vi "SGDRegressor.vi"(8 "error in":errorcluster) -> (0 "error out":errorcluster, 3 "out":refnum<class "SGDRegressor.lvclass">)   [LabVIEW 2020]
doc: "Linear model fitted by minimizing a regularized empirical loss with SGD\n\n SGD stands for Stochastic Gradient Descent: the gradient of the loss is\n estimated each sample at a time and the model is updated along the way with\n a decreasing strength schedule (aka learning rate).\n\n The regularizer is a penalty added to the loss function that shrinks model\n parameters towards the zero vector using either the squared euclidean norm\n L2 or the absolute norm L1 or a combination of both (Elastic Net). If the\n parameter update crosses the 0.0 value because of the regularizer, the\n update is truncated to 0.0 to allow for learning sparse models and achieve\n online feature selection.\n\n This implementation works with data represented as dense numpy arrays of\n floating point values for the features.\n\n Read more in the :ref:`User Guide <sgd>`.\n\n Parameters\n ----------\n loss : str, default='squared_loss'\n The loss function to be used. The possible values are 'squared_loss',\n 'huber', 'epsilon_insensitive', or 'squared_epsilon_insensitive'\n\n The 'squared_loss' refers to the ordinary least squares fit.\n 'huber' modifies 'squared_loss' to focus less on getting outliers\n correct by switching from squared to linear loss past a distance of\n epsilon. 'epsilon_insensitive' ignores errors less than epsilon and is\n linear past that; this is the loss function used in SVR.\n 'squared_epsilon_insensitive' is the same but becomes squared loss past\n a tolerance of epsilon.\n\n More details about the losses formulas can be found in the\n :ref:`User Guide <sgd_mathematical_formulation>`.\n\n penalty : {'l2', 'l1', 'elasticnet'}, default='l2'\n The penalty (aka regularization term) to be used. Defaults to 'l2'\n which is the standard regularizer for linear SVM models. 'l1' and\n 'elasticnet' might bring sparsity to the model (feature selection)\n not achievable with 'l2'.\n\n alpha : float, default=0.0001\n Constant that multiplies the regularization term. The higher the\n value, the stronger the regularization.\n Also used to compute the learning rate when set to `learning_rate` is\n set to 'optimal'.\n\n l1_ratio : float, default=0.15\n The Elastic Net mixing parameter, with 0 <= l1_ratio <= 1.\n l1_ratio=0 corresponds to L2 penalty, l1_ratio=1 to L1.\n Only used if `penalty` is 'elasticnet'.\n\n fit_intercept : bool, default=True\n Whether the intercept should be estimated or not. If False, the\n data is assumed to be already centered.\n\n max_iter : int, default=1000\n The maximum number of passes over the training data (aka epochs).\n It only impacts the behavior in the ``fit`` method, and not the\n :meth:`partial_fit` method.\n\n .. versionadded:: 0.19\n\n tol : float, default=1e-3\n The stopping criterion. If it is not None, training will stop\n when (loss > best_loss - tol) for ``n_iter_no_change`` consecutive\n epochs.\n Convergence is checked against the training loss or the\n validation loss depending on the `early_stopping` parameter.\n\n .. versionadded:: 0.19\n\n shuffle : bool, default=True\n Whether or not the training data should be shuffled after each epoch.\n\n verbose : int, default=0\n The verbosity level.\n\n epsilon : float, default=0.1\n Epsilon in the epsilon-insensitive loss functions; only if `loss` is\n 'huber', 'epsilon_insensitive', or 'squared_epsilon_insensitive'.\n For 'huber', determines the threshold at which it becomes less\n important to get the prediction exactly right.\n For epsilon-insensitive, any differences between the current prediction\n and the correct label are ignored if they are less than this threshold.\n\n random_state : int, RandomState instance, default=None\n Used for shuffling the data, when ``shuffle`` is set to ``True``.\n Pass an int for reproducible output across multiple function calls.\n See :term:`Glossary <random_state>`.\n\n learning_rate : string, default='invscaling'\n The learning rate schedule:\n\n - 'constant': `eta = eta0`\n - 'optimal': `eta = 1.0 / (alpha * (t + t0))`\n where t0 is chosen by a heuristic proposed by Leon Bottou.\n - 'invscaling': `eta = eta0 / pow(t, power_t)`\n - 'adaptive': eta = eta0, as long as the training keeps decreasing.\n Each time n_iter_no_change consecutive epochs fail to decrease the\n training loss by tol or fail to increase validation score by tol if\n early_stopping is True, the current learning rate is divided by 5.\n\n .. versionadded:: 0.20\n Added 'adaptive' option\n\n eta0 : double, default=0.01\n The initial learning rate for the 'constant', 'invscaling' or\n 'adaptive' schedules. The default value is 0.01.\n\n power_t : double, default=0.25\n The exponent for inverse scaling learning rate.\n\n early_stopping : bool, default=False\n Whether to use early stopping to terminate training when validation\n score is not improving. If set to True, it will automatically set aside\n a fraction of training data as validation and terminate\n training when validation score returned by the `score` method is not\n improving by at least `tol` for `n_iter_no_change` consecutive\n epochs.\n\n .. versionadded:: 0.20\n Added 'early_stopping' option\n\n validation_fraction : float, default=0.1\n The proportion of training data to set aside as validation set for\n early stopping. Must be between 0 and 1.\n Only used if `early_stopping` is True.\n\n .. versionadded:: 0.20\n Added 'validation_fraction' option\n\n n_iter_no_change : int, default=5\n Number of iterations with no improvement to wait before stopping\n fitting.\n Convergence is checked against the training loss or the\n validation loss depending on the `early_stopping` parameter.\n\n .. versionadded:: 0.20\n Added 'n_iter_no_change' option\n\n warm_start : bool, default=False\n When set to True, reuse the solution of the previous call to fit as\n initialization, otherwise, just erase the previous solution.\n See :term:`the Glossary <warm_start>`.\n\n Repeatedly calling fit or partial_fit when warm_start is True can\n result in a different solution than when calling fit a single time\n because of the way the data is shuffled.\n If a dynamic learning rate is used, the learning rate is adapted\n depending on the number of samples already seen. Calling ``fit`` resets\n this counter, while ``partial_fit`` will result in increasing the\n existing counter.\n\n average : bool or int, default=False\n When set to True, computes the averaged SGD weights accross all\n updates and stores the result in the ``coef_`` attribute. If set to\n an int greater than 1, averaging will begin once the total number of\n samples seen reaches `average`. So ``average=10`` will begin\n averaging after seeing 10 samples.\n\n Attributes\n ----------\n coef_ : ndarray of shape (n_features,)\n Weights assigned to the features.\n\n intercept_ : ndarray of shape (1,)\n The intercept term.\n\n average_coef_ : ndarray of shape (n_features,)\n Averaged weights assigned to the features. Only available\n if ``average=True``.\n\n .. deprecated:: 0.23\n Attribute ``average_coef_`` was deprecated\n in version 0.23 and will be removed in 1.0 (renaming of 0.25).\n\n average_intercept_ : ndarray of shape (1,)\n The averaged intercept term. Only available if ``average=True``.\n\n .. deprecated:: 0.23\n Attribute ``average_intercept_`` was deprecated\n in version 0.23 and will be removed in 1.0 (renaming of 0.25).\n\n n_iter_ : int\n The actual number of iterations before reaching the stopping criterion.\n\n t_ : int\n Number of weight updates performed during training.\n Same as ``(n_iter_ * n_samples)``.\n\n \nAvailable methods:\nGet Attributes\nGet Params\nSet Params"
uses:
  SGDRegressor.lvclass
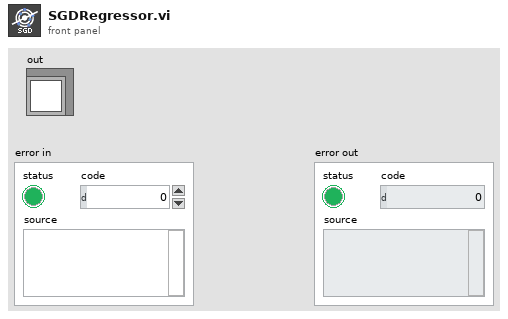
[diagram p1: front panel]
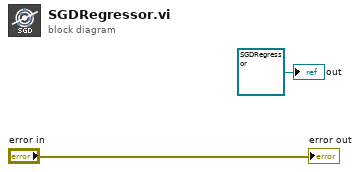
[diagram p0: block diagram]
diagram:
  "out" <- refnum<class "SGDRegressor.lvclass"> refnum ("model")
  "error out" <- "error in"
